vi "Set Graph Legend.vi"(0 "XYGraph in":refnum<vi>, 5 "Active Plot":i32, 7 "Plot Name":string, 9 "# Plots":i32, 11 "error in (no error)":errorcluster, 12 "Plot Style":T1={"Plot Style"=enum."unchanged", "Histogram Type"=enum."Left Bound", "Line Tickness"=enum."unchanged", "Line Style"=enum."unchanged", "Point Style"=enum."unchanged", "Line Color"=0, "Point Color"=0, "Anti-aliased"=FALSE, "Line Color Chooser"=enum."unchanged", "Point Color Chooser"=enum."unchanged", "Line Color List"="", "Point Color List"=""}) -> (15 "error out":errorcluster)   [LabVIEW 2019, in "Histogram Window.lvlib"]
uses:
  Histogram Window.lvlib
  Plot Style 3.ctl
  XY Graph Add-Ons.lvlib
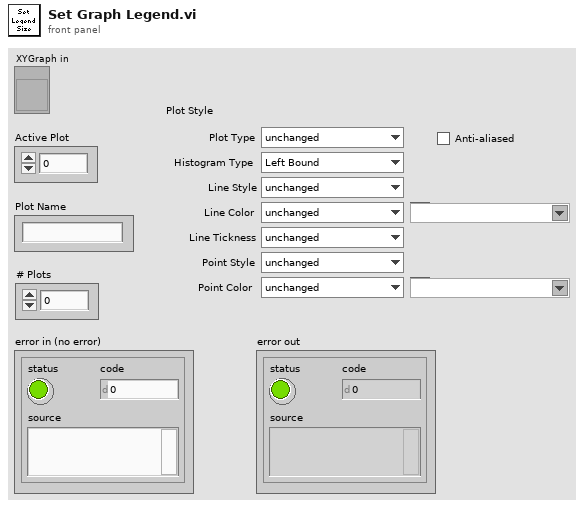
[diagram p1: front panel]
types:
  T1 = typedef "Plot Style 3.ctl" = cluster{"Plot Style":enum16{"unchanged", "Line", "Symbol", "Line + Symbol", "Histogram", "Histogram + Symbol"}, "Histogram Type":enum16{"unchanged", "Left Bound", "Center", "Right Bound"}, "Line Tickness":enum16{"unchanged", "Thin", "1 pixel", "2 pixel", "3 pixel", "4 pixel", "5 pixel"}, "Line Style":enum16{"unchanged", "Plain", "Long Dash", "Short Dash", "Long-Short Dash", "Long-Short-Short Dash"}, "Point Style":enum16{"unchanged", "None", "Empty Circle", "Filled Circle", "Thick Circle", "Dotted Circle", "Empty Square", "Filled Square", "Thick Square", "Dotted Square", "Small Filled Square", "Dot", "Cross", "Tiny Cross", "Large X", "Small x", "Diamond", "Small Empty Square"}, "Line Color":u32, "Point Color":u32, "Anti-aliased":bool, "Line Color Chooser":enum16{"unchanged", "Color Box", "Color List"}, "Point Color Chooser":enum16{"unchanged", "Color Box", "Color List"}, "Line Color List":string, "Point Color List":string}
  T2 = typedef "Single Plot Style 2.ctl" = cluster{"Plot Style":enum16{"unchanged", "Line", "Symbol", "Line + Symbol", "Histogram", "Histogram + Symbol"}, "Histogram Type":enum16{"unchanged", "Left Bound", "Center", "Right Bound"}, "Line Tickness":enum16{"unchanged", "Thin", "1 pixel", "2 pixel", "3 pixel", "4 pixel", "5 pixel"}, "Line Style":enum16{"unchanged", "Plain", "Long Dash", "Short Dash", "Long-Short Dash", "Long-Short-Short Dash"}, "Point Style":enum16{"unchanged", "None", "Empty Circle", "Filled Circle", "Thick Circle", "Dotted Circle", "Empty Square", "Filled Square", "Thick Square", "Dotted Square", "Small Filled Square", "Dot", "Cross", "Tiny Cross", "Large X", "Small x", "Diamond", "Small Empty Square"}, "Line Color":u32, "Line Color defined?":bool, "Point Color":u32, "Point Color defined?":bool, "Anti-aliased":bool}
  T3 = typedef "XY Graph Add-Ons.lvlib/XY Graph Refnum.ctl" = refnum<vi>
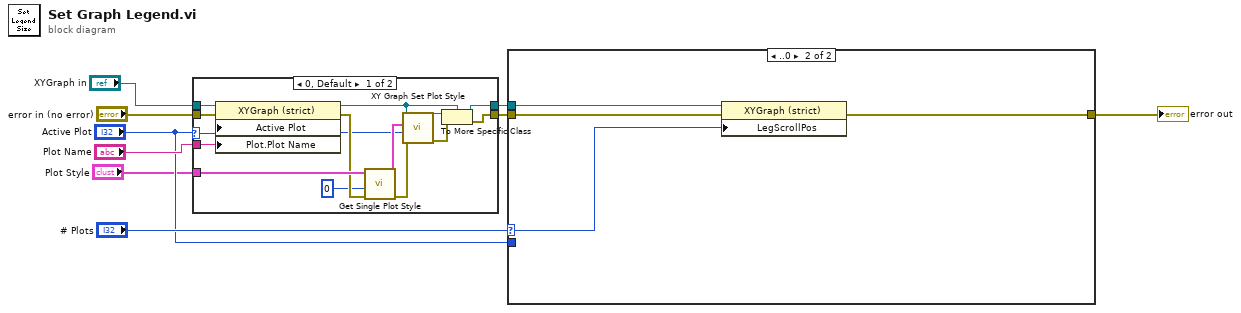
[diagram p0: block diagram]
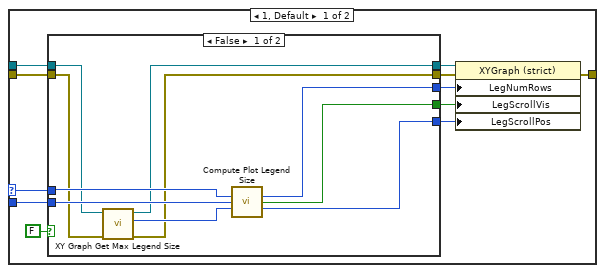
[diagram p2: hidden frame]
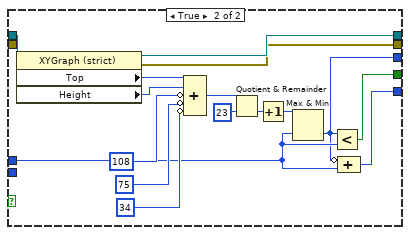
[diagram p3: hidden frame]
diagram:
  n1 = case shown="0, Default" "Active Plot" {
    selector: "Active Plot" -> [w10 _]
    tunnel: "error in (no error)" -> [w23 w24]
    tunnel: "Plot Name" -> [w22 _]
    tunnel: "XYGraph in" -> [w21 w25]
    tunnel: [w19 w25] -> w6
    tunnel: [w16 w24] -> w5
    tunnel: "Plot Style" -> [w15 _]
    frame 0, Default {
      n2 = property on="Property Node" class="XYGraph (strict)"(reference=w21, error in=w23, "Active Plot"=w10, "Plot.Plot Name"=w22) -> (reference out=w18:refnum<vi>, error out=w14:errorcluster)
      n3 = call "Get Single Plot Style.vi"("Error In"=w14, "index"=0, "Plot Style in"=w15) -> ("Error Out"=w13:errorcluster, "Plot Style out"=w11:T2)  [unwired: 7 in]
      n4 = call "XY Graph Set Plot Style.vi"("Error In"=w13, "Plot Index (0)"=w10, "Single Plot Style"=w11, "XY Graph Refnum in"=w18) -> ("Error Out"=w17:errorcluster, "XY Graph Refnum out"=w20:refnum<vi>)  [unwired: 6 in]
      n5 = To More Specific Class(target class=w18, reference=w20, error in=w17) -> (specific class reference=w19:refnum<vi>, error out=w16:errorcluster)
    }
    frame -1 {
    }
  }
  n6 = case shown="..0" "# Plots" {
    selector: "# Plots" -> [w30 w64]
    tunnel: w6 -> [w36 w67]
    tunnel: w5 -> [w33 w66]
    tunnel: [w35 w65] -> w4
    tunnel: "Active Plot" -> [w26 _]
    frame 1, Default {
      n7 = case shown="False" FALSE {
        tunnel: w36 -> [w39 w63]
        tunnel: [w38 w62] -> w34
        tunnel: w33 -> [w40 w61]
        tunnel: [w37 w60] -> w32
        tunnel: [w44 w50] -> w31
        tunnel: w30 -> [w46 w49]
        tunnel: [w45 w48] -> w29
        tunnel: [w43 w47] -> w28
        tunnel: w26 -> [w42 _]
        frame False {
          n8 = call "XY Graph Get Max Legend Size.vi"("Error In"=w40, "XYGraph Refnum"=w39) -> ("Error Out"=w37:errorcluster, "Max Legend Size"=w41:i32, "XYGraph Refnum"=w38:T3)  [unwired: 6 in, 1 out]
          n9 = call "Compute Plot Legend Size.vi"("# Plots"=w46, "Current Plot (Last)"=w42, "Max Legend Size"=w41) -> ("LegNumRows"=w45:u32, "LegScrollVis"=w44:bool, "LegScrollPos"=w43:u32)  [unwired: 10 in]
        }
        frame True {
          n10 = property class="XYGraph (strict)"(reference=w63, error in=w61) -> (reference out=w62:refnum<vi>, error out=w60:errorcluster, "Top"=w59:i32, "Height"=w58:u32)
          n11 = Compound Arithmetic op=ADD(w59, w58, invert u32 108 ("value"), invert u32 75 ("value"), invert u32 34 ("value")) -> (w54:u32)
          n12 = Quotient & Remainder(x=w54, y=u32 23) -> (floor(x/y)=w52:u32)  [unwired: 1 out]
          n13 = Increment(x=w52) -> (x+1=w51:u32)
          n14 = Max & Min(x=w51, y=w49) -> (min(x,y)=w48:u32)  [unwired: 1 out]
          n15 = Less?(x=w48, y=w49) -> (x < y?=w50:bool)
          n16 = Compound Arithmetic op=ADD(invert w48, w49) -> (w47:u32)
        }
      }
      n17 = property on="Property Node" class="XYGraph (strict)"(reference=w34, error in=w32, "LegNumRows"=w29, "LegScrollVis"=w31, "LegScrollPos"=w28) -> (error out=w35:errorcluster)  [unwired: 1 out]
    }
    frame ..0 {
      n18 = property on="Property Node" class="XYGraph (strict)"(reference=w67, error in=w66, "LegScrollPos"=w64) -> (error out=w65:errorcluster)  [unwired: 1 out]
    }
  }
  "error out" <- w4
